vi "Read S11.vi"(7 "Timeout [ms]":u32=2000, 8 "Error In":errorcluster, 10 "Channel (1)":i32=1 caption="Channel", 11 "VISA Refnum In":refnum<visa-resource-name>) -> (0 "Error Out":errorcluster, 1 "S11":T2 {"Z" format="%#_4g"}, 2 "Frequency span":T1, 3 "VISA Refnum Out":refnum<visa-resource-name>)   [LabVIEW 2016]
uses:
  Processing/Trace (cplx).ctl
  <vilib>/Analysis/NI_AALBase.lvlib
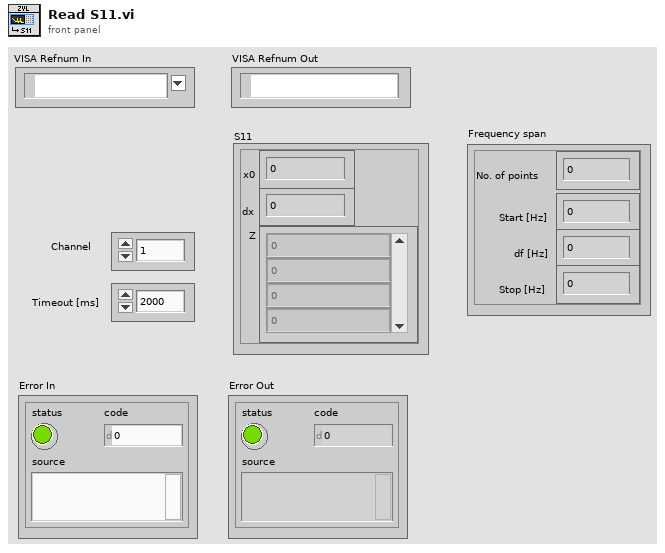
[diagram p1: front panel]
types:
  T1 = cluster{"Start [Hz]":dbl, "No. of points":i32, "df [Hz]":dbl, "Stop [Hz]":dbl}
  T2 = typedef "Trace (cplx).ctl" = cluster{"x0":dbl, "dx":dbl, "Z":cdb[]}
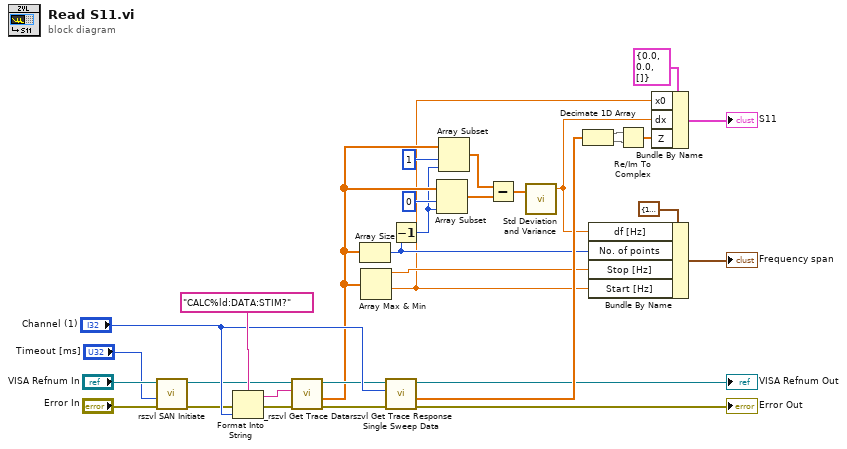
[diagram p0: block diagram]
diagram:
  n1 = call <instrlib>:"rszvl SAN Initiate.vi"("error in (no error)"="Error In", "Timeout (15000)"="Timeout [ms]", "VISA resource name"="VISA Refnum In") -> ("error out"=w15:errorcluster, "VISA resource name out"=w18:refnum<visa-resource-name>)  [unwired: 7 in]
  n2 = Format Into String(format string="CALC%ld:DATA:STIM?", error in=w15, "Channel (1)") -> (resulting string=w21:string, error out=w14:errorcluster)  [unwired: 1 in]
  n3 = call <instrlib>:"_rszvl Get Trace Data.vi"("error in (no error)"=w14, "Command"=w21, "VISA resource name"=w18) -> ("error out"=w16:errorcluster, "Amplitude"=w9:dbl[])  [unwired: 6 in, 1 out]
  n4 = Array Size(array=w9) -> (size(s)=w4:i32)
  n5 = Array Max & Min(array=w9) -> (max value=w5:dbl, min value=w3:dbl)  [unwired: 2 out]
  n6 = call <instrlib>:"rszvl Get Trace Response Single Sweep Data.vi"("error in (no error)"=w16, "Channel (1)"="Channel (1)", "VISA resource name"=w18) -> ("error out"=→"Error Out":errorcluster, "Trace Data"=w26:dbl[], "VISA resource name out"=→"VISA Refnum Out":refnum<visa-resource-name>)  [unwired: 6 in]
  n7 = Decrement(x=w4) -> (x-1=w8:i32)
  n8 = Array Subset(array=w9, index=0, length=w8) -> (w10:dbl[])
  n9 = Array Subset(array=w9, index=1, length=w8) -> (w11:dbl[])
  n10 = Subtract(x=w11, y=w10) -> (x-y=w7:dbl[])
  n11 = call <vilib>:"Std Deviation and Variance.vi"("X"=w7) -> ("mean"=w2:dbl)  [unwired: 1 in, 2 out]
  n12 = Decimate 1D Array(w26) -> (w24:dbl[], w23:dbl[])
  n13 = Bundle By Name(cluster=T1 {"Start [Hz]"=1000000.0, "No. of points"=10, "df [Hz]"=1.0, "Stop [Hz]"=2000000.0} ("Frequency span"), "df [Hz]"=w2, "No. of points"=w4, "Stop [Hz]"=w5, "Start [Hz]"=w3) -> (→"Frequency span":T1)
  n14 = Re/Im To Complex(1:w23, 2:w24) -> (0:w22:cdb[])
  n15 = Bundle By Name(cluster=T2 {"x0"=0.0, "dx"=0.0, "Z"=[]} ("S11"), "x0"=w3, "dx"=w2, "Z"=w22) -> (→"S11":T2)
